vi "IR Sensor.vi"(6 "Offset Y":cluster{"Offset Y L":dbl, "Offset Y R":dbl}={"Offset Y L"=15.0, "Offset Y R"=15.0}, 7 "Array trans":dbl[][](array[numeric])=[[0.566, 100.0], [0.627, 90.0], [0.71, 80.0], [0.761, 70.0], [0.803, 65.0], [0.86, 60.0], [0.9, 55.0], [0.958, 50.0], [0.98, 46.0], [1.015, 42.0], [1.035, 36.0], [1.0534, 30.0], [1.09, 26.0], [1.13, 24.0], [1.23, 22.0], [1.32, 20.0], [1.38, 19.0], [1.46, 18.0], [1.52, 17.0], [1.6, 16.0], [1.69, 15.0], [1.78, 14.0], [1.89, 13.0], [2.04, 12.0], [2.2, 11.0], [2.4, 10.0], [2.6, 9.0], [2.834, 8.0], [3.1, 7.0], [3.13, 6.0]], 8 "error in (no error)":errorcluster, 11 "Analog In in":T2) -> (0 "error out":errorcluster, 2 "IR":cluster{"IR Left":dbl, "IR Right":dbl}, 3 "Analog In out":T1)   [LabVIEW 2020]
uses:
  <vilib>/High Genius/HG_WSI_Tookit/Dependencies/Library/Analog In/Analog In.lvclass
  C:/Program Files (x86)/National Instruments/LabVIEW 2020/vi.lib/High Genius/HG_WSI_Tookit/Dependencies/Library/HG_LIB/HG_LIB.lvclass
  <vilib>/High Genius/HG_WSI_Tookit/Dependencies/Library/HG_LIB/HG_LIB.lvclass/HG_LIB.ctl
  <vilib>/High Genius/HG_WSI_Tookit/Dependencies/Library/HG_LIB/HG_LIB.lvclass
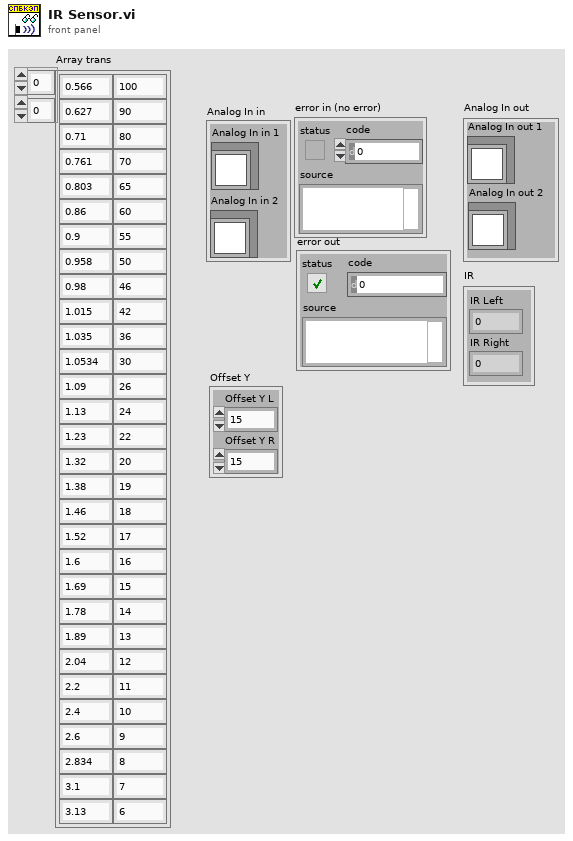
[diagram p1: front panel]
types:
  T1 = cluster{"Analog In out 1":refnum<class "Analog In.lvclass">, "Analog In out 2":refnum<class "Analog In.lvclass">}
  T2 = cluster{"Analog In in 1":refnum<class "Analog In.lvclass">, "Analog In in 2":refnum<class "Analog In.lvclass">}
  T3 = cluster{"data":cluster{"ai22":sgl, "ai23":sgl, "ai24":sgl, "ai25":sgl, "pulse12":i32, "pulse13":i32, "pwm14":i32, "pwm15":i32, "pwm16":i32, "do17":bool, "do18":bool, "do19":bool, "do20":bool, "do21":bool, "di11":bool, "di9":bool, "motor0":u8, "motor1":u8, "motor2":u8, "motor3":u8, "dir00":u8, "dir01":u8, "dir02":u8, "dir03":u8, "dir10":u8, "dir11":u8, "dir12":u8, "dir13":u8, "limit0":bool, "limit1":bool, "limit2":bool, "limit3":bool, "limit4":bool, "limit5":bool, "limit6":bool, "limit7":bool, "lsb0H":u8, "lsb1H":u8, "lsb2H":u8, "lsb3H":u8, "lsb0L":u8, "lsb1L":u8, "lsb2L":u8, "lsb3L":u8, "enc0_counters":u32, "enc1_counters":u32, "enc2_counters":u32, "enc3_counters":u32, "counter10":u32, "counter8":u32, "reset_enc0":bool, "reset_enc1":bool, "reset_enc2":bool, "reset_enc3":bool, "pitch":sgl, "roll":sgl, "yaw":sgl, "zero_yaw":bool}}
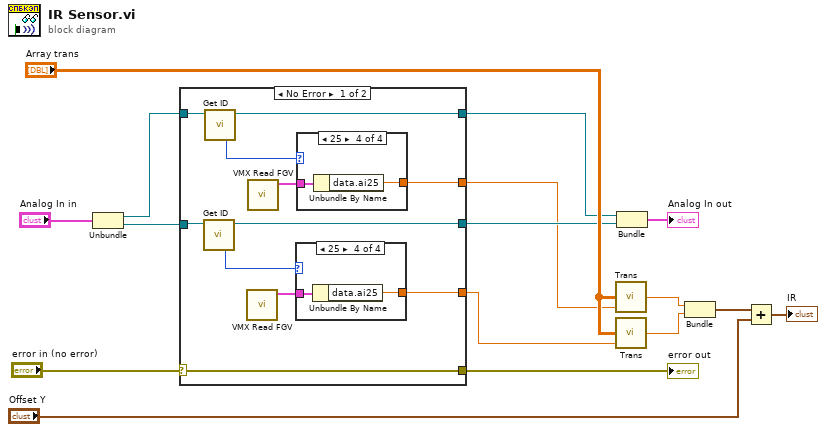
[diagram p0: block diagram]
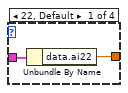
[diagram p2: hidden frame]
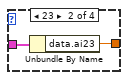
[diagram p3: hidden frame]
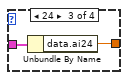
[diagram p4: hidden frame]
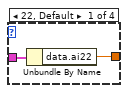
[diagram p5: hidden frame]
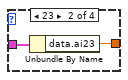
[diagram p6: hidden frame]
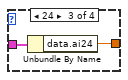
[diagram p7: hidden frame]
diagram:
  n1 = Unbundle("Analog In in") -> ("Analog In in 1"=w1:refnum<class "Analog In.lvclass">, "Analog In in 2"=w3:refnum<class "Analog In.lvclass">)
  n2 = case shown="No Error" "error in (no error)" {
    selector: "error in (no error)" -> [w23 w46]
    tunnel: [w23 w46] -> w7
    tunnel: [w27 w45] -> w4
    tunnel: w1 -> [w22 w45]
    tunnel: [w24 _] -> w2
    tunnel: w3 -> [w19 w44]
    tunnel: [w18 _] -> w6
    tunnel: [w17 w44] -> w5
    frame No Error {
      n3 = call <vilib>:"Get ID.vi"("HG_LIB in"=w19) -> ("ID"=w21:u32, "HG_LIB out"=w17:refnum<class "Analog In.lvclass">)  [unwired: 9 in]
      n4 = call <vilib>:"Get ID.vi"("HG_LIB in"=w22) -> ("ID"=w25:u32, "HG_LIB out"=w27:refnum<class "Analog In.lvclass">)  [unwired: 9 in]
      n5 = call <vilib>:"VMX Read FGV.vi"() -> ("Read Data"=w20:T3)  [unwired: 10 in, 1 out]
      n6 = call <vilib>:"VMX Read FGV.vi"() -> ("Read Data"=w26:T3)  [unwired: 10 in, 1 out]
      n7 = case shown="25" w21 {
        tunnel: w20 -> [w29 w31 w32 w35]
        tunnel: [w28 w30 w33 w34] -> w18
        frame 22, Default {
          n8 = Unbundle By Name(w29) -> ("data.ai22"=w28:sgl)
        }
        frame 23 {
          n9 = Unbundle By Name(w31) -> ("data.ai23"=w30:sgl)
        }
        frame 24 {
          n10 = Unbundle By Name(w32) -> ("data.ai24"=w33:sgl)
        }
        frame 25 {
          n11 = Unbundle By Name(w35) -> ("data.ai25"=w34:sgl)
        }
      }
      n12 = case shown="25" w25 {
        tunnel: w26 -> [w37 w39 w40 w43]
        tunnel: [w36 w38 w41 w42] -> w24
        frame 22, Default {
          n13 = Unbundle By Name(w37) -> ("data.ai22"=w36:sgl)
        }
        frame 23 {
          n14 = Unbundle By Name(w39) -> ("data.ai23"=w38:sgl)
        }
        frame 24 {
          n15 = Unbundle By Name(w40) -> ("data.ai24"=w41:sgl)
        }
        frame 25 {
          n16 = Unbundle By Name(w43) -> ("data.ai25"=w42:sgl)
        }
      }
    }
    frame Error {
    }
  }
  "error out" <- w7
  n17 = call "Trans.vi"("Y"=w2, "Array 4"="Array trans") -> ("Y value"=w13:dbl)  [unwired: 1 in]
  n18 = call "Trans.vi"("Y"=w6, "Array 4"="Array trans") -> ("Y value"=w12:dbl)  [unwired: 1 in]
  n19 = Bundle("Analog In in 1"=w4, "Analog In in 2"=w5) -> (→"Analog In out":T2)  [unwired: 1 in]
  n20 = Bundle("Y value"=w13, "Y value"=w12) -> (w10:cluster{"Y value":dbl, "Y value":dbl})  [unwired: 1 in]
  n21 = Add(x=w10, y="Offset Y") -> (x+y=→"IR":cluster{dbl, dbl})
